vi "SetValueAuto.vi"(0 "VI Reference In":refnum<vi>, 2 "delimiter (>>)":string=">>", 5 "Control Path":string, 7 "Value (Signaling)":variant, 11 "error in":errorcluster) -> (4 "VI Reference Out":refnum<vi>, 15 "error out":errorcluster)   [LabVIEW 2016, in "Drona.lvlib" / "ControlValue.lvlib"]
doc: "Sets the value of control which is specified. \n\nThe input control name is given as a string , incase of path, use delimiters inbetween the path."
uses:
  ControlValue.lvlib
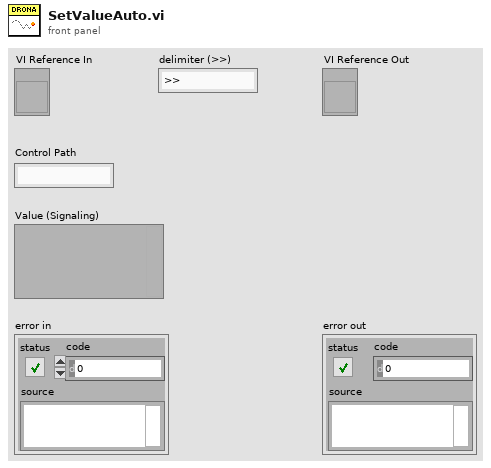
[diagram p1: front panel]
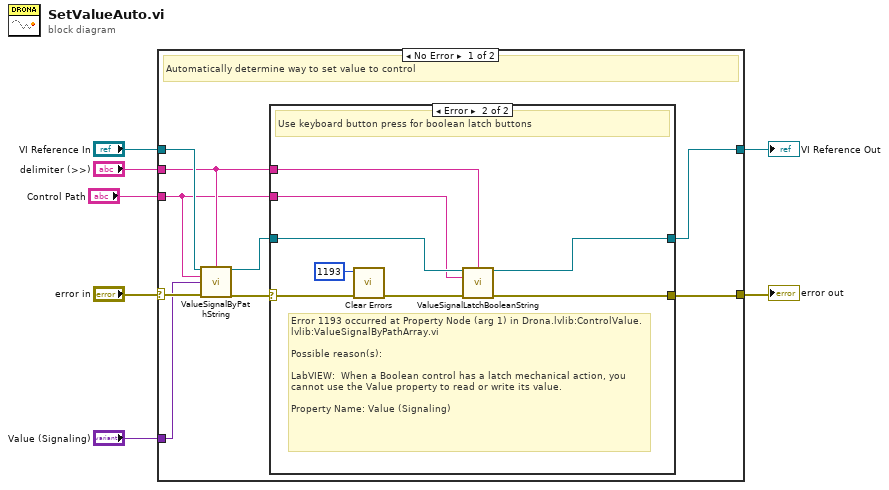
[diagram p0: block diagram]
diagram:
  n1 = case shown="No Error" "error in" {
    selector: "error in" -> [w16 w28]
    tunnel: "Control Path" -> [w10 _]
    tunnel: "VI Reference In" -> [w15 w27]
    tunnel: [w9 w27] -> w4
    tunnel: "Value (Signaling)" -> [w14 _]
    tunnel: [w8 w28] -> w2
    tunnel: "delimiter (>>)" -> [w11 _]
    frame No Error {
      # "Automatically determine way to set value to control"
      n2 = call "ValueSignalByPathString.vi"("VI Reference In"=w15, "delimiter (>>)"=w11, "Control Path"=w10, "Value (Signaling)"=w14, "error in"=w16) -> ("VI Reference Out"=w12:refnum<vi>, "error out"=w13:errorcluster)  [unwired: 9 in]
      n3 = case shown="Error" w13 {
        selector: w13 -> [w17 w26]
        tunnel: w12 -> [w18 w25]
        tunnel: w11 -> [_ w24]
        tunnel: w10 -> [_ w23]
        tunnel: [w18 w22] -> w9
        tunnel: [w17 w21] -> w8
        frame No Error {
        }
        frame Error {
          # "Error 1193 occurred at Property Node (arg 1) in Drona.lvlib:ControlValue.lvlib:ValueSignalByPathArray.vi\n\nPossible reason(s):\n\nLabVIEW:  When a Boolean control has a latch mechanical action, you cannot use the Value property to read or write its value.\n\nProperty Name: Value (Signaling)"
          # "Use keyboard button press for boolean latch buttons"
          n4 = call <vilib>:"Clear Errors.vi"("error in (no error)"=w26, "specific error code to clear (0: all)"=1193) -> ("error out"=w20:errorcluster)  [unwired: 4 in, 1 out]
          n5 = call "ValueSignalLatchBooleanString.vi"("VI Reference In"=w25, "delimiter (>>)"=w24, "Control Path"=w23, "error in"=w20) -> ("VI Reference Out"=w22:refnum<vi>, "error out"=w21:errorcluster)  [unwired: 10 in]
        }
      }
    }
    frame Error {
    }
  }
  "error out" <- w2
  "VI Reference Out" <- w4
